vi "VISP CRC32 (String).vi"(10 "crc32 in (0)":u32 format="%08x", 11 "String in":string) -> (3 "crc32 out":u32 format="%08x")   [LabVIEW 2019, in "VI Snippet.lvlib"]
doc: "Calculates the cyclic redundancy check 32-bit (CRC32) for PNG chunks from the <b>String in</b>.\n\nCreated by: Ryan Pacini"
uses:
  VI Snippet.lvlib
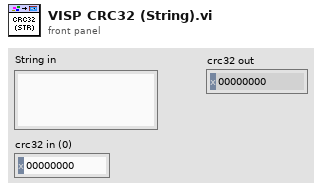
[diagram p1: front panel]
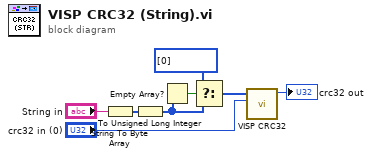
[diagram p0: block diagram]
diagram:
  n1 = String To Byte Array(string="String in") -> (unsigned byte array=w7:u8[])
  n2 = To Unsigned Long Integer(number=w7) -> (unsigned 32bit integer=w5:u32[])
  n3 = Empty Array?(array=w5) -> (empty?=w4:bool)
  n4 = Select(t=u32[] [0] ("Data in"), s=w4, f=w5) -> (s? t:f=w1:u32[])
  n5 = call "VISP CRC32.vi"("crc32 in (0)"="crc32 in (0)", "Data in"=w1) -> ("crc32 out"=→"crc32 out":u32)  [unwired: 9 in]
